vi "Control Panel.vi"   [LabVIEW 2023]
uses:
  Power Supply/Power Supply.lvclass
  Level Meter/Level Meter.lvclass
  Temperature Controller/Temperature Controller.lvclass
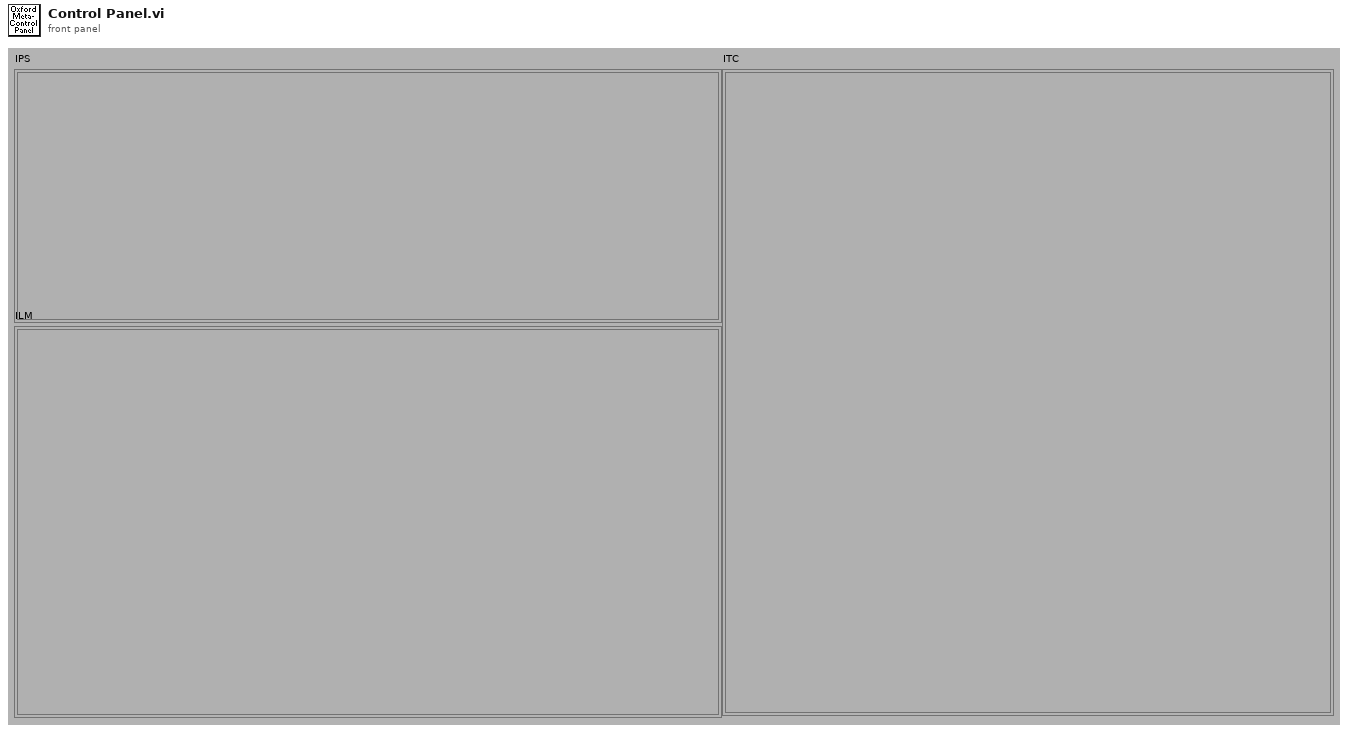
[diagram p1: front panel]
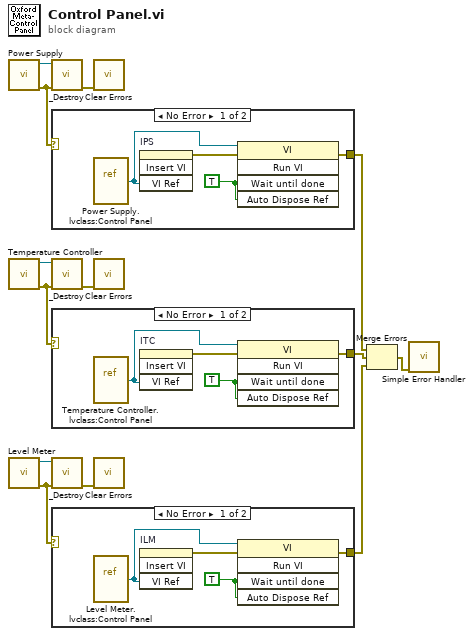
[diagram p0: block diagram]
diagram:
  n1 = call "Power Supply.vi"() -> ("error out"=w9:errorcluster, "Power Supply out"=w8:refnum<class "Power Supply.lvclass">)  [unwired: 10 in]
  n2 = call "Temperature Controller.vi"() -> ("error out"=w13:errorcluster, "Temperature Controller out"=w12:refnum<class "Temperature Controller.lvclass">)  [unwired: 10 in]
  n3 = call "Level Meter.vi"() -> ("error out"=w10:errorcluster, "Level Meter out"=w11:refnum<class "Level Meter.lvclass">)  [unwired: 10 in]
  n4 = call-dynamic "_Destroy.vi"("error in (no error)"=w9, "Instrument in"=w8) -> ("error out"=w3:errorcluster)  [unwired: 9 in]
  n5 = case shown="No Error" w9 {
    tunnel: [w14 _] -> w5
    frame No Error {
      w17 = TRUE ("Wait Until Done")
      n6 = vi-ref "Power Supply.lvclass:Control Panel.vi"() -> (w16:refnum<vi>)
      n7 = invoke on="IPS" class="SubPanel" method="Insert VI"("VI Ref"=w16) -> (error out=w15:errorcluster)  [unwired: 3 in, 3 out]
      n8 = invoke class="VI" method="Run VI"(reference=w16, error in=w15, "Wait until done"=w17, "Auto Dispose Ref"=w17) -> (error out=w14:errorcluster)  [unwired: 1 in, 4 out]
    }
    frame Error {
    }
  }
  n9 = call-dynamic "_Destroy.vi"("error in (no error)"=w13, "Instrument in"=w12) -> ("error out"=w2:errorcluster)  [unwired: 9 in]
  n10 = case shown="No Error" w13 {
    tunnel: [w18 _] -> w6
    frame No Error {
      w21 = TRUE ("Wait Until Done")
      n11 = vi-ref "Temperature Controller.lvclass:Control Panel.vi"() -> (w20:refnum<vi>)
      n12 = invoke on="ITC" class="SubPnl" method="Insert VI"("VI Ref"=w20) -> (error out=w19:errorcluster)  [unwired: 3 in, 3 out]
      n13 = invoke class="VI" method="Run VI"(reference=w20, error in=w19, "Wait until done"=w21, "Auto Dispose Ref"=w21) -> (error out=w18:errorcluster)  [unwired: 1 in, 4 out]
    }
    frame Error {
    }
  }
  n14 = call-dynamic "_Destroy.vi"("error in (no error)"=w10, "Instrument in"=w11) -> ("error out"=w1:errorcluster)  [unwired: 9 in]
  n15 = case shown="No Error" w10 {
    tunnel: [w22 _] -> w7
    frame No Error {
      w23 = TRUE ("Wait Until Done")
      n16 = vi-ref "Level Meter.lvclass:Control Panel.vi"() -> (w25:refnum<vi>)
      n17 = invoke on="ILM" class="SubPnl" method="Insert VI"("VI Ref"=w25) -> (error out=w24:errorcluster)  [unwired: 3 in, 3 out]
      n18 = invoke class="VI" method="Run VI"(reference=w25, error in=w24, "Wait until done"=w23, "Auto Dispose Ref"=w23) -> (error out=w22:errorcluster)  [unwired: 1 in, 4 out]
    }
    frame Error {
    }
  }
  n19 = call <vilib>:"Clear Errors.vi"("error in (no error)"=w3) -> ()  [unwired: 5 in, 2 out]
  n20 = call <vilib>:"Clear Errors.vi"("error in (no error)"=w2) -> ()  [unwired: 5 in, 2 out]
  n21 = call <vilib>:"Clear Errors.vi"("error in (no error)"=w1) -> ()  [unwired: 5 in, 2 out]
  n22 = Merge Errors(w5, w6, w7) -> (w4:errorcluster)
  n23 = call <vilib>:"Simple Error Handler.vi"("error in (no error)"=w4) -> ()  [unwired: 4 in, 5 out]
